vi "test network stream.vi"() -> ()   [LabVIEW 2017]
panel:
  out "Data out":fxp<+/-,17,5>[](array[numeric]) format="%#_17g"
  in  "Data to write":fxp<+/-,17,5>[](array[numeric]) format="%#_17g"
  in  "IP":string
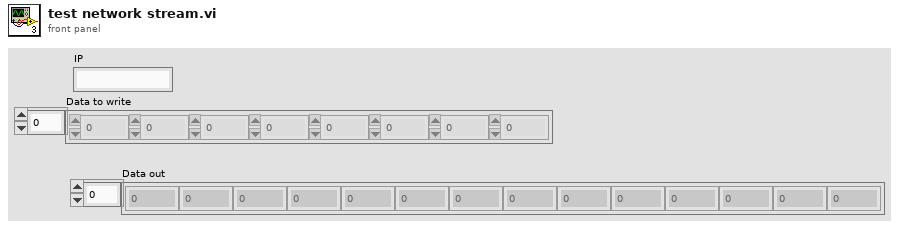
[diagram p1: front panel]
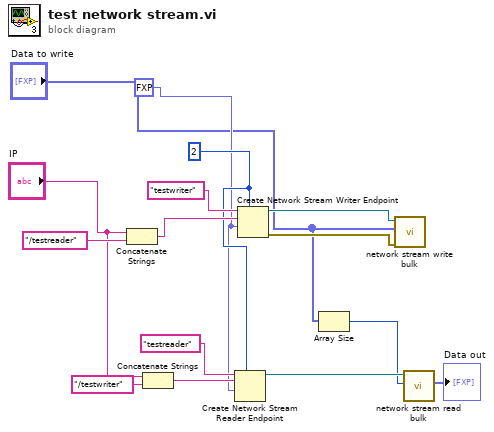
[diagram p0: block diagram]
diagram:
  w5 = fxp<+/-,17,5> 0.0 ("Data")
  w8 = 2 ("writer buffer size")
  n1 = Concatenate Strings("IP", "/testreader" ("string")) -> (w14:string)
  n2 = Concatenate Strings("IP", "/testwriter" ("string")) -> (w10:string)
  n3 = Create Network Stream Reader Endpoint(7:w8, 9:w5, 10:w10, 11:"testreader" ("reader name")) -> (3:w4:refnum<k21>)  [unwired: 3 in, 1 out]
  n4 = Create Network Stream Writer Endpoint(7:w8, 9:w5, 10:w14, 11:"testwriter" ("writer name")) -> (0:w6:errorcluster, 3:w7:refnum<k21>)  [unwired: 3 in]
  n5 = Array Size(array="Data to write") -> (size(s)=w2:i32)
  n6 = call "network stream write bulk.vi"("error in (no error)"=w6, "Data"="Data to write", "endpoint in"=w7) -> ()  [unwired: 7 in, 2 out]
  n7 = call "network stream read bulk.vi"("endpoint in"=w4, "Data num"=w2) -> ("Data"=→"Data out":fxp<+/-,17,5>[])  [unwired: 6 in, 2 out]
